vi "Timer.vi"() -> ()   [LabVIEW 2015]
panel:
  in  "RestTime":dbl=60.0
  out "Time":dbl format="%.2f"
  out "Record?":bool
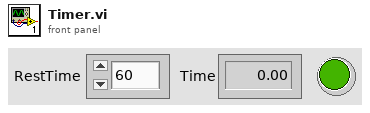
[diagram p1: front panel]
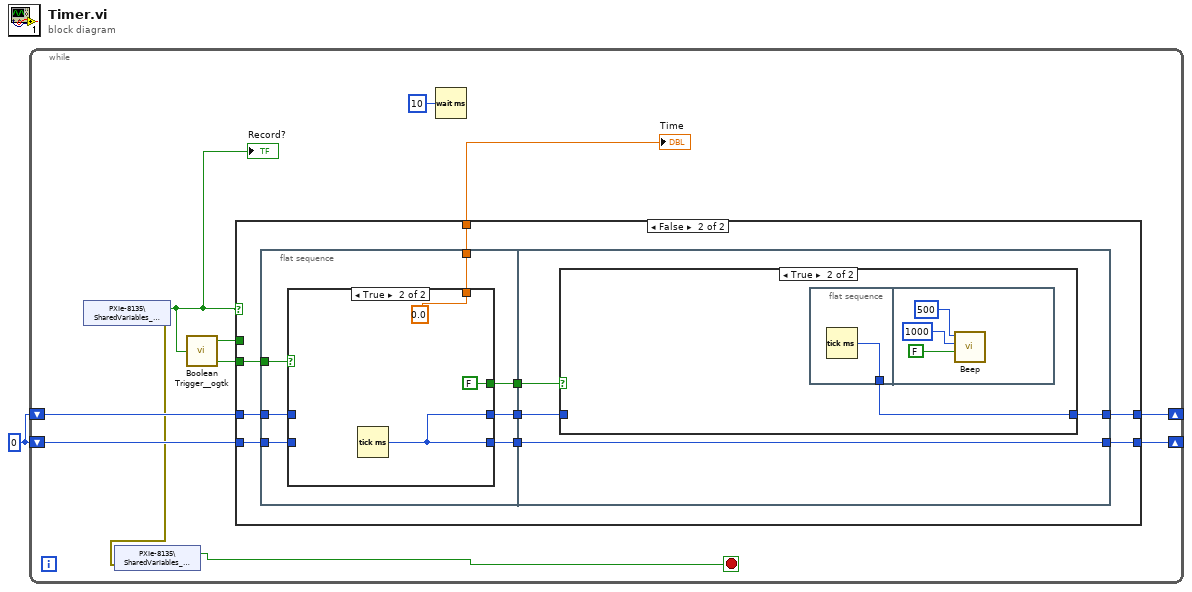
[diagram p0: block diagram]
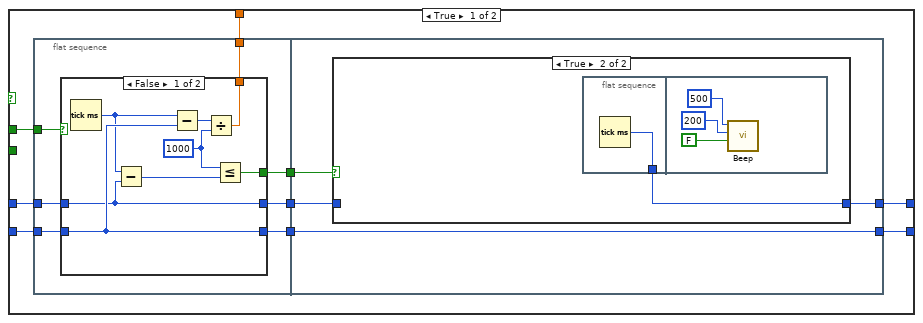
[diagram p2: hidden frame]
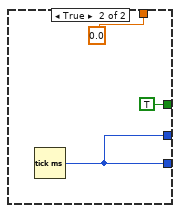
[diagram p3: hidden frame]
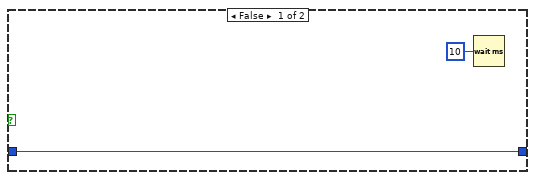
[diagram p4: hidden frame]
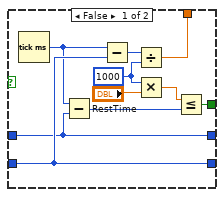
[diagram p5: hidden frame]
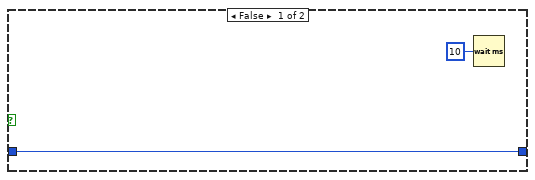
[diagram p6: hidden frame]
diagram:
  w1 = u32 0 ("millisecond timer value")
  n1 = while {
    shift-right: [w10] -> _
    shift-left: w1 -> [w9]
    shift-right: [w7] -> _
    shift-left: w1 -> [w6]
    stop <- w3 stop-if-true
    n2 = shared-variable "PXIe-8135\\SharedVariables_Network.lvlib\\Record?"() -> (w12:bool, error out=w2:errorcluster)  [unwired: 1 in]
    "Record?" <- w12
    n3 = shared-variable "PXIe-8135\\SharedVariables_Network.lvlib\\Stop RT"(error in=w2) -> (w3:bool)  [unwired: 1 out]
    n4 = call <userlib>:"Boolean Trigger__ogtk.vi"("Boolean Input"=w12) -> ("Rising Edge"=w11:bool, "Falling Edge"=w4:bool)  [unwired: 1 in]
    n5 = case shown="False" w12 {
      tunnel: w11 -> [w21 _]
      tunnel: [w20 w59] -> w10
      tunnel: w9 -> [w18 w57]
      tunnel: [w17 w56] -> w8
      tunnel: [w16 w55] -> w7
      tunnel: w6 -> [w14 w53]
      tunnel: w4 -> [_ w51]
      frame True {
        n6 = flat-sequence {
          tunnel: w21 -> [w28]
          tunnel: [w27] -> w19
          tunnel: w18 -> [w26]
          tunnel: [w25] -> w17
          tunnel: [w24] -> w15
          tunnel: w14 -> [w23]
          tunnel: [w22] -> w13
          tunnel: [w43] -> w20
          tunnel: w19 -> [w43]
          tunnel: [w42] -> w16
          tunnel: w15 -> [w41]
          tunnel: w13 -> [w40]
          frame #0 {
            n7 = case shown="False" w28 {
              tunnel: [w36 w38] -> w27
              tunnel: w26 -> [w36 _]
              tunnel: [w33 0.0] -> w25
              tunnel: [w29 w38] -> w24
              tunnel: w23 -> [w29 _]
              tunnel: [w30 TRUE] -> w22
              frame False {
                w31 = u32 1000 ("y")
                n8 = Tick Count (ms)() -> (millisecond timer value=w34:u32)
                n9 = Subtract(x=w34, y=w29) -> (x-y=w32:u32)
                n10 = Subtract(x=w34, y=w36) -> (x-y=w35:u32)
                n11 = Divide(x=w35, y=w31) -> (x/y=w33:dbl)
                n12 = Less Or Equal?(x=w31, y=w32) -> (x <= y?=w30:bool)
              }
              frame True {
                n13 = Tick Count (ms)() -> (millisecond timer value=w38:u32)
              }
            }
          }
          frame #1 {
            n14 = case shown="True" w40 {
              tunnel: [w44 w46] -> w42
              tunnel: w41 -> [w44 _]
              frame False {
                n15 = Wait (ms)(milliseconds to wait=u32 10) -> ()  [unwired: 1 out]
              }
              frame True {
                n16 = flat-sequence {
                  tunnel: [w47] -> w46
                  frame #0 {
                    n17 = Tick Count (ms)() -> (millisecond timer value=w47:u32)
                  }
                  frame #1 {
                    n18 = call <vilib>:"Beep.vi"("use system alert? (T)"=FALSE, "duration (msec)"=u32 200, "frequency (Hz)"=u32 500) -> ()  [unwired: 9 in]
                  }
                }
              }
            }
          }
        }
      }
      frame False {
        n19 = flat-sequence {
          tunnel: [w66] -> w58
          tunnel: w57 -> [w65]
          tunnel: [w64] -> w56
          tunnel: [w63] -> w54
          tunnel: w53 -> [w62]
          tunnel: [w61] -> w52
          tunnel: w51 -> [w60]
          tunnel: [w83] -> w59
          tunnel: w58 -> [w83]
          tunnel: [w82] -> w55
          tunnel: w54 -> [w81]
          tunnel: w52 -> [w80]
          frame #0 {
            n20 = case shown="True" w60 {
              tunnel: [w76 w78] -> w66
              tunnel: w65 -> [w76 _]
              tunnel: [w73 0.0] -> w64
              tunnel: [w70 w78] -> w63
              tunnel: w62 -> [w70 _]
              tunnel: [w71 FALSE] -> w61
              frame False {
                w68 = u32 1000 ("y")
                n21 = Tick Count (ms)() -> (millisecond timer value=w74:u32)
                n22 = Subtract(x=w74, y=w70) -> (x-y=w72:u32)
                n23 = Subtract(x=w74, y=w76) -> (x-y=w75:u32)
                n24 = Divide(x=w75, y=w68) -> (x/y=w73:dbl)
                n25 = Multiply(x=w68, y="RestTime") -> (x*y=w67:dbl)
                n26 = Less Or Equal?(x=w67, y=w72) -> (x <= y?=w71:bool)
              }
              frame True {
                n27 = Tick Count (ms)() -> (millisecond timer value=w78:u32)
              }
            }
          }
          frame #1 {
            n28 = case shown="True" w80 {
              tunnel: [w84 w86] -> w82
              tunnel: w81 -> [w84 _]
              frame False {
                n29 = Wait (ms)(milliseconds to wait=u32 10) -> ()  [unwired: 1 out]
              }
              frame True {
                n30 = flat-sequence {
                  tunnel: [w87] -> w86
                  frame #0 {
                    n31 = Tick Count (ms)() -> (millisecond timer value=w87:u32)
                  }
                  frame #1 {
                    n32 = call <vilib>:"Beep.vi"("use system alert? (T)"=FALSE, "duration (msec)"=u32 1000, "frequency (Hz)"=u32 500) -> ()  [unwired: 9 in]
                  }
                }
              }
            }
          }
        }
      }
    }
    "Time" <- w8
    n33 = Wait (ms)(milliseconds to wait=u32 10) -> ()  [unwired: 1 out]
  }
